vi "indicator.vi"() -> ()   [LabVIEW 2023]
panel:
  in  "stop":bool
  out "Numeric":dbl
  in  "入力値（少数）":dbl(slide) scale=0.0..10.0
  in  "Tab Control":enum32{"少数", "整数"}(tab)
  out "Side Progress":dbl(slide) scale=0.0..10.0
  out "Side Grad":dbl(slide) scale=0.0..10.0
  out "Meter":dbl(knob) scale=0.0..10.0
  out "Gauge":dbl(knob) scale=0.0..10.0
  out "Tank":dbl(slide) scale=0.0..10.0
  out "Progress":dbl(slide) scale=0.0..10.0
  out "Thermometer":dbl(slide) scale=0.0..10.0
  out "Grad":dbl(slide) scale=0.0..10.0
  out "Side Progress 2":i32(slide) scale=0.0..10.0
  out "Side Grad 2":i32(slide) scale=0.0..10.0
  out "Meter 2":i32(knob) scale=0.0..10.0
  out "Gauge 2":i32(knob) scale=0.0..10.0
  out "Tank 2":i32(slide) scale=0.0..10.0
  out "Progress  2":i32(slide) scale=0.0..10.0
  out "Thermometer 2":i32(slide) scale=0.0..10.0
  out "Grad 2":i32(slide) scale=0.0..10.0
  # "Express内のNum  lndsのアイコンの動きを知るためのVIです。\nDBL（少数を含む）とi32（整数）２種類の型で表示確認できます。\nプログラム終了したい場合STOPボタンを押してください"
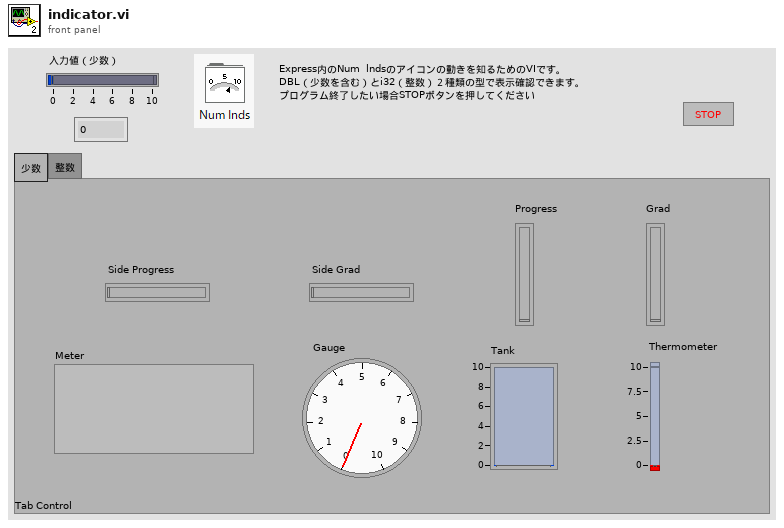
[diagram p1: front panel]
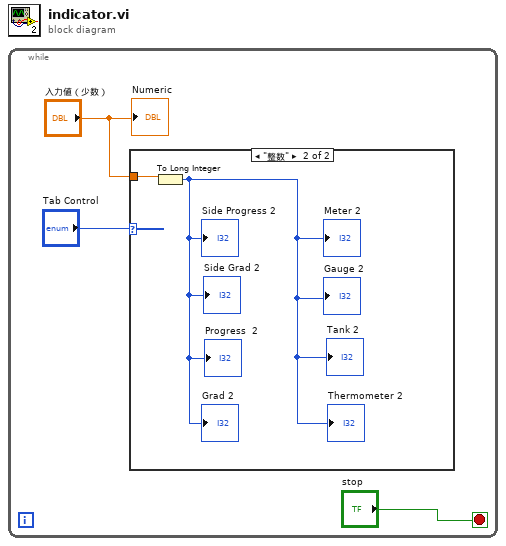
[diagram p0: block diagram]
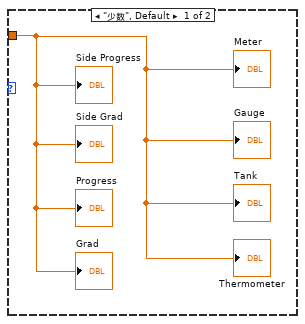
[diagram p2: hidden frame]
diagram:
  n1 = while {
    stop <- "stop" stop-if-true
    n2 = case shown="\"整数\"" "Tab Control" {
      tunnel: "入力値（少数）" -> [w4 w6]
      frame "少数", Default {
        "Side Grad" <- w4
        "Side Progress" <- w4
        "Progress" <- w4
        "Grad" <- w4
        "Meter" <- w4
        "Gauge" <- w4
        "Tank" <- w4
        "Thermometer" <- w4
      }
      frame "整数" {
        n3 = To Long Integer(number=w6) -> (32bit integer=→"Progress  2" →"Grad 2" →"Side Grad 2" →"Side Progress 2" →"Gauge 2" →"Meter 2" →"Tank 2" →"Thermometer 2":i32)
      }
    }
    "Numeric" <- "入力値（少数）"
  }
